vi "Flatten UIP Value.vi"(11 "CaptionUIP In":refnum<class "CaptionUIP.lvclass">) -> (0 "Error Out":errorcluster, 2 "String Value":string, 3 "CaptionUIP Out":refnum<class "CaptionUIP.lvclass">)   [LabVIEW 2020, in "UIM.lvlib" / "CaptionUIP.lvclass"]
uses:
  CaptionUIP.lvclass
  CaptionUIP.lvclass/CaptionUIP.ctl
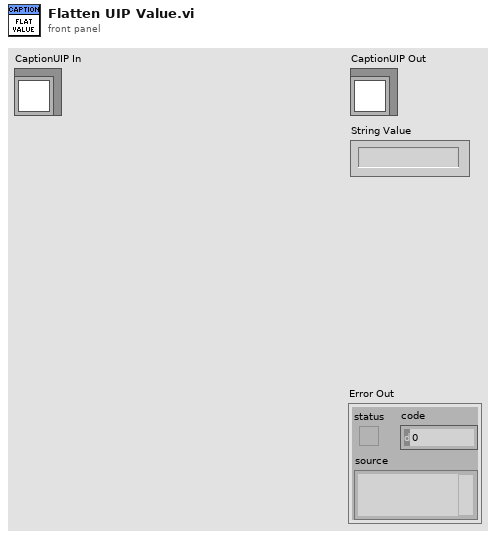
[diagram p1: front panel]
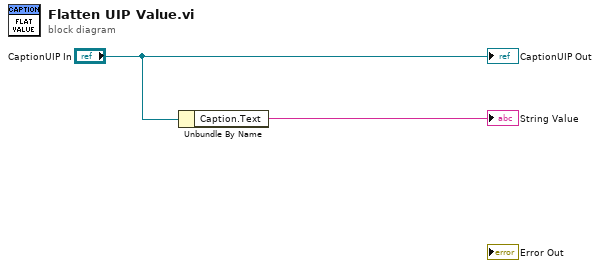
[diagram p0: block diagram]
diagram:
  n1 = Unbundle By Name("CaptionUIP In") -> ("Caption.Text"=→"String Value":string)
  "CaptionUIP Out" <- "CaptionUIP In"
